vi "picoSetChannel.vi"(8 "error in (no error)":errorcluster, 9 "Channel B Settings":T1, 10 "Channel A Settings":T1, 11 "Handle Out":i16) -> (0 "error out":errorcluster, 3 "Handle Out":i16)   [LabVIEW 2011]
uses:
  PS2000a.dll
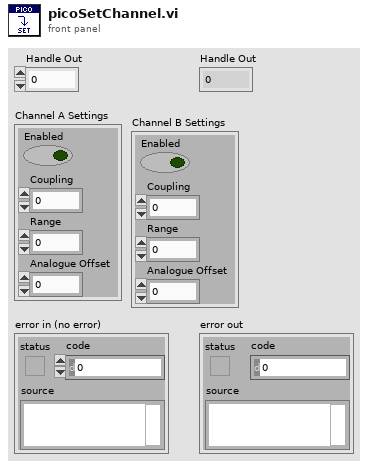
[diagram p1: front panel]
types:
  T1 = cluster{"Enabled":bool, "Coupling":i16, "Range":u16, "Analogue Offset":sgl}
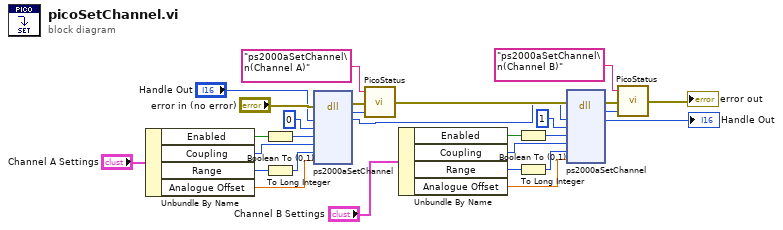
[diagram p0: block diagram]
diagram:
  n1 = Unbundle By Name("Channel A Settings") -> ("Enabled"=w22:bool, "Coupling"=w19:i16, "Range"=w24:u16, "Analogue Offset"=w20:sgl)
  n2 = Boolean To (0,1)(Boolean=w22) -> (0, 1=w21:i16)
  n3 = To Long Integer(number=w24) -> (32bit integer=w23:i32)
  n4 = dll-call lib="ps2000a.dll" fn="ps2000aSetChannel" ("ps2000a.dll:_ps3000_open_unit@0")(error in="error in (no error)", "handle"="Handle Out", "channel"=0, "enabled"=w21, "dc"=w19, "range"=w23, "analogueOffset"=w20) -> (error out=w17:errorcluster, "PICO_STATUS"=w18:u32, "handle"=w1:i16)  [unwired: 7 in, 1 out]
  n5 = call "PicoStatus.vi"("PICO STATUS"=w18, "error in"=w17, "source"="ps2000aSetChannel\n(Channel A)") -> ("error out"=w4:errorcluster)
  n6 = Unbundle By Name("Channel B Settings") -> ("Enabled"=w9:bool, "Coupling"=w12:i16, "Range"=w7:u16, "Analogue Offset"=w11:sgl)
  n7 = Boolean To (0,1)(Boolean=w9) -> (0, 1=w10:i16)
  n8 = To Long Integer(number=w7) -> (32bit integer=w8:i32)
  n9 = dll-call lib="ps2000a.dll" fn="ps2000aSetChannel" ("ps2000a.dll:_ps3000_open_unit@0")(error in=w4, "handle"=w1, "channel"=1, "enabled"=w10, "dc"=w12, "range"=w8, "analogueOffset"=w11) -> (error out=w14:errorcluster, "PICO_STATUS"=w13:u32, "handle"=→"Handle Out":i16)  [unwired: 7 in, 1 out]
  n10 = call "PicoStatus.vi"("PICO STATUS"=w13, "error in"=w14, "source"="ps2000aSetChannel\n(Channel B)") -> ("error out"=→"error out":errorcluster)
